vi "Close Wfm Sessions.vi"(8 "Error In":errorcluster, 11 "Async State Vars":T1) -> (0 "Error Out":errorcluster)   [LabVIEW 2014, in "Waveform-Processing-Custom-Device Engine.lvlib"]
uses:
  Waveform-Processing-Custom-Device Engine.lvlib
  Types/Async State Vars.ctl
  Types/Async FIFOs.ctl
  <vilib>/NI Veristand/Custom Device Waveform API/Single Waveform Read (DBL)/Single Waveform Read (DBL).lvclass
  <vilib>/NI Veristand/Custom Device Waveform API/Single Waveform Write (DBL)/Single Waveform Write (DBL).lvclass
  <vilib>/NI Veristand/Custom Device API/Waveform Data Reference.ctl
  <vilib>/NI Veristand/Custom Device Waveform API/Single Waveform Read (DBL)/NI VeriStand - Close Single Waveform Read Session (DBL).vi
  <vilib>/NI Veristand/Custom Device Waveform API/Single Waveform Write (DBL)/NI VeriStand - Close Single Waveform Write Session (DBL).vi
  <vilib>/NI Veristand/Custom Device Waveform API/NI_VS Custom Device Waveform API.lvlib
  <vilib>/NI Veristand/Custom Device API/Custom Device API.lvlib
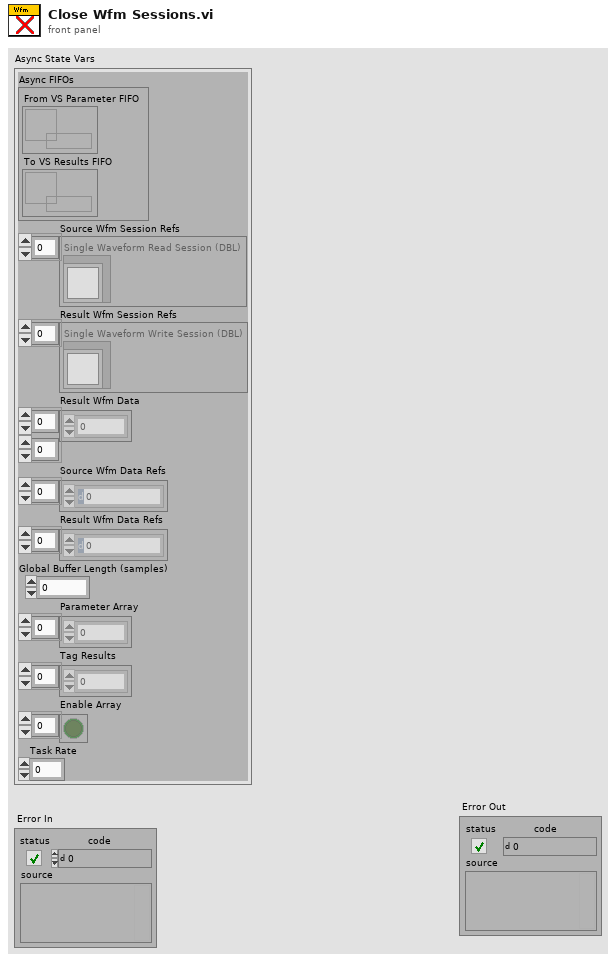
[diagram p1: front panel]
types:
  T1 = typedef "Waveform-Processing-Custom-Device Engine.lvlib/Async State Vars.ctl" = cluster{"Async FIFOs":T2, "Source Wfm Session Refs":refnum<class "Single Waveform Read (DBL).lvclass">[], "Result Wfm Session Refs":refnum<class "Single Waveform Write (DBL).lvclass">[], "Result Wfm Data":dbl[][], "Source Wfm Data Refs":T3[], "Result Wfm Data Refs":T3[], "Global Buffer Length (samples)":dbl, "Parameter Array":dbl[], "Tag Results":dbl[], "Enable Array":bool[], "Task Rate":dbl}
  T2 = typedef "Waveform-Processing-Custom-Device Engine.lvlib/Async FIFOs.ctl" = cluster{"From VS Parameter FIFO":refnum<k33>, "To VS Results FIFO":refnum<k33>}
  T3 = typedef "Custom Device API.lvlib/Waveform Data Reference.ctl" = i32
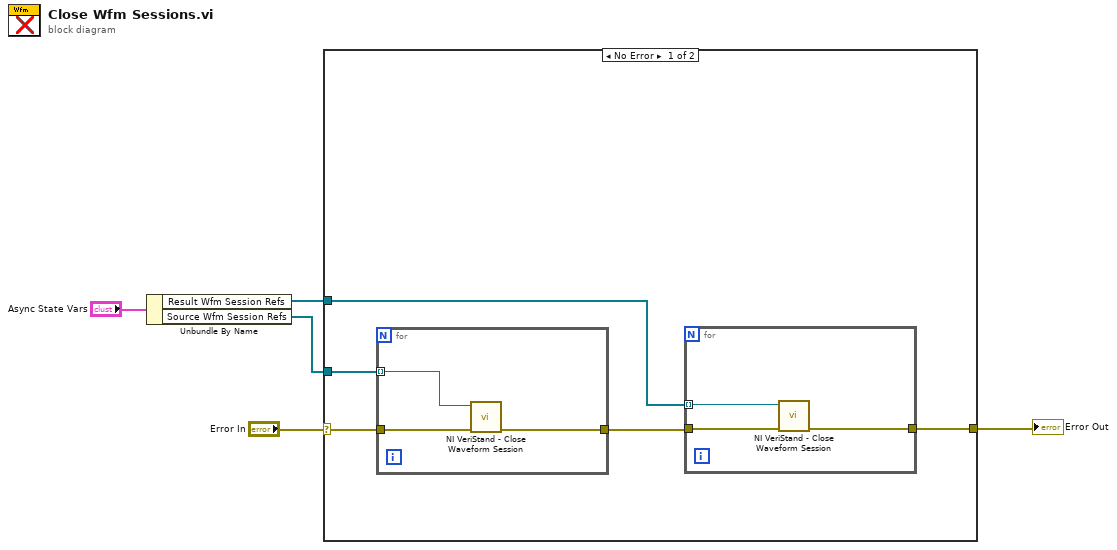
[diagram p0: block diagram]
diagram:
  n1 = Unbundle By Name("Async State Vars") -> ("Result Wfm Session Refs"=w2:refnum<class "Single Waveform Write (DBL).lvclass">[], "Source Wfm Session Refs"=w1:refnum<class "Single Waveform Read (DBL).lvclass">[])
  n2 = case shown="No Error" "Error In" {
    selector: "Error In" -> [w10 w17]
    tunnel: [w8 w17] -> w4
    tunnel: w2 -> [w6 _]
    tunnel: w1 -> [w7 _]
    frame No Error {
      n3 = for {
        tunnel: w10 -> [w16]
        tunnel: [w15] -> w9
        tunnel: w7 -> [w14] mode=indexing
        n4 = call-poly <vilib>:"NI VeriStand - Close Waveform Session.vi"("error in (no error)"=w16, "Single Waveform Read Session (DBL)"=w14) -> ("error out"=w15:errorcluster)  [unwired: 9 in]
      }
      n5 = for {
        tunnel: w9 -> [w13]
        tunnel: [w12] -> w8
        tunnel: w6 -> [w11] mode=indexing
        n6 = call-poly <vilib>:"NI VeriStand - Close Waveform Session.vi"("error in (no error)"=w13, "Single Waveform Write Session (DBL)"=w11) -> ("error out"=w12:errorcluster)  [unwired: 9 in]
      }
    }
    frame Error {
    }
  }
  "Error Out" <- w4
